vi "subNodes Colour up.vi"(0 "GObjects[]":refnum<vi>[](array[refnum]), 5 "Parent Color":u32(colorbox), 7 "Default Colour (White)":u32(colorbox)=16448250, 9 "Defined Colour (YellowLight)":u32(colorbox)=16711615, 11 "error in (no error)":errorcluster) -> (15 "error out":errorcluster)   [LabVIEW 2020, in "ColourUpStructures.lvlib"]
doc: "Colour Up all Structures in <b>GObjects[]</b> Array."
uses:
  ColourUpStructures.lvlib
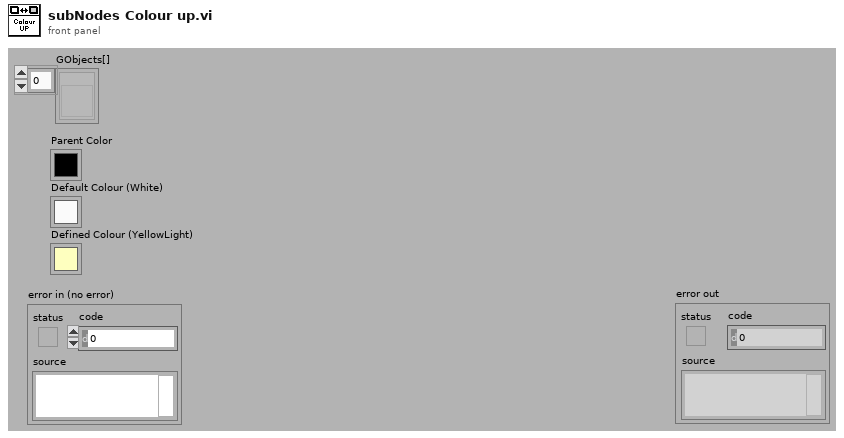
[diagram p1: front panel]
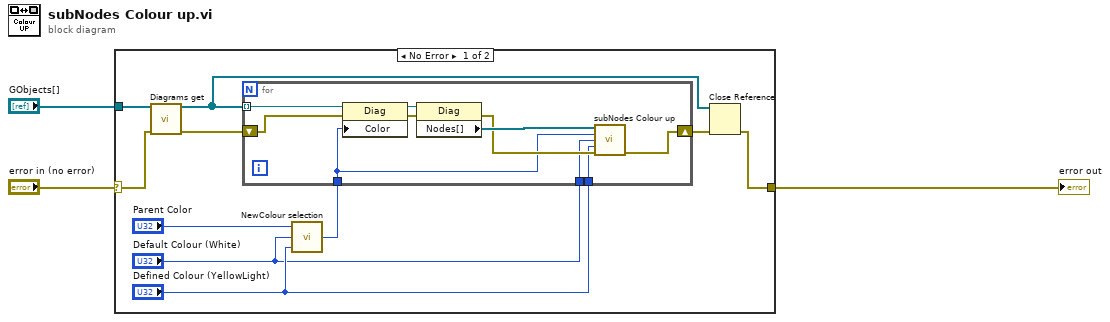
[diagram p0: block diagram]
diagram:
  n1 = case shown="No Error" "error in (no error)" {
    selector: "error in (no error)" -> [w12 w24]
    tunnel: "GObjects[]" -> [w13 _]
    tunnel: [w8 w24] -> w1
    frame No Error {
      n2 = call "Diagrams get.vi"("GObjects[]"=w13, "error in (no error)"=w12) -> ("Diagrams[]"=w9:refnum<vi>[], "error out"=w11:errorcluster)  [unwired: 12 in]
      n3 = call "NewColour selection.vi"("Defined Colour"="Defined Colour (YellowLight)", "Default Colour"="Default Colour (White)", "Old Color"="Parent Color") -> ("New Colour"=w6:u32)
      n4 = for {
        tunnel: w9 -> [w23] mode=indexing
        shift-right: [w17] -> w10
        shift-left: w11 -> [w22]
        tunnel: w6 -> [w14]
        tunnel: "Defined Colour (YellowLight)" -> [w16]
        tunnel: "Default Colour (White)" -> [w15]
        n5 = property class="Diag"(reference=w23, error in=w22, "Color"=w14) -> (reference out=w21:refnum<vi>, error out=w20:errorcluster)
        n6 = property class="Diag"(reference=w21, error in=w20) -> (error out=w18:errorcluster, "Nodes[]"=w19:refnum<vi>[])  [unwired: 1 out]
        n7 = call "subNodes Colour up.vi"("GObjects[]"=w19, "Parent Color"=w14, "Default Colour (White)"=w15, "Defined Colour (YellowLight)"=w16, "error in (no error)"=w18) -> ("error out"=w17:errorcluster)  [unwired: 10 in]
      }
      n8 = Close Reference(reference=w9, error in (no error)=w10) -> (error out=w8:errorcluster)
    }
    frame Error {
    }
  }
  "error out" <- w1
